vi "Part 1.vi"(11 "Input":string) -> (3 "Output":i64)   [LabVIEW 2021]
uses:
  <userlib>/_OpenG.lib/string/string.llb/Convert EOLs (String)__ogtk.vi
panel:
  out "Array":i64[](array[numeric])
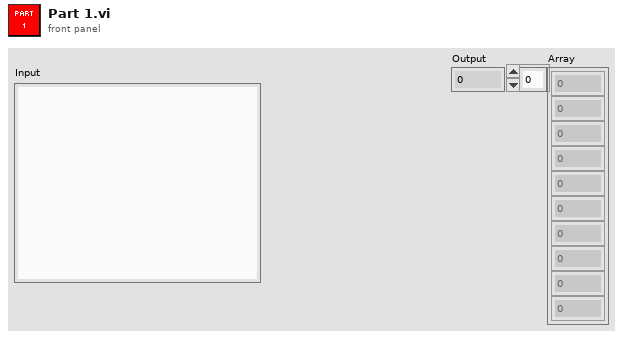
[diagram p1: front panel]
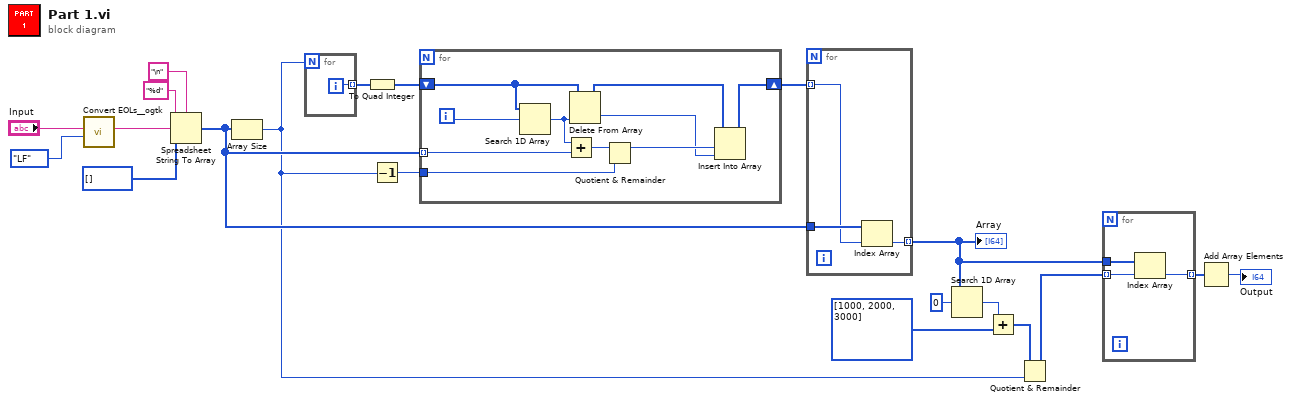
[diagram p0: block diagram]
diagram:
  n1 = call-poly <userlib>:"Convert EOLs__ogtk.vi"("Convert to:"=enum16{"CR", "LF", "CRLF"}."LF", "String in"="Input") -> ("String out"=w16:string)  [unwired: 9 in]
  n2 = Spreadsheet String To Array(delimiter (Tab)="\n", format string="%d", spreadsheet string=w16, array type (2D Dbl)=i64[] []) -> (array=w12:i64[])
  n3 = Array Size(array=w12) -> (size(s)=w8:i32)
  n4 = for {
    N: w8 -> [_]
    tunnel: [w21] -> w7 mode=indexing
    i -> [w21]
  }
  n5 = To Quad Integer(1:w7) -> (0:w6:i64[])
  n6 = Decrement(x=w8) -> (x-1=w14:i32)
  n7 = for {
    tunnel: w12 -> [w31] mode=indexing
    shift-right: [w23] -> w5
    shift-left: w6 -> [w25]
    tunnel: w14 -> [w22]
    i -> [w27]
    n8 = Search 1D Array(1D array=w25, element=w27) -> (index of element=w30:i32)  [unwired: 1 in]
    n9 = Add(x=w30, y=w31) -> (x+y=w29:i64)
    n10 = Delete From Array(array=w25, index=w30) -> (deleted portion=w26:i64, array with subset deleted=w24:i64[])  [unwired: 1 in]
    n11 = Quotient & Remainder(x=w29, y=w22) -> (x-y*floor(x/y)=w28:i64)  [unwired: 1 out]
    n12 = Insert Into Array(array=w24, index=w28, new element=w26) -> (w23:i64[])
  }
  n13 = for {
    tunnel: w5 -> [w33] mode=indexing
    tunnel: w12 -> [w34]
    tunnel: [w32] -> w1 mode=indexing
    n14 = Index Array(array=w34, index=w33) -> (element=w32:i64)
  }
  "Array" <- w1
  n15 = Search 1D Array(1D array=w1, element=i64 0) -> (index of element=w4:i32)  [unwired: 1 in]
  n16 = Add(x=w4, y=i64[] [1000, 2000, 3000]) -> (x+y=w3:i64[])
  n17 = Quotient & Remainder(x=w3, y=w8) -> (x-y*floor(x/y)=w2:i64[])  [unwired: 1 out]
  n18 = for {
    tunnel: w1 -> [w37]
    tunnel: w2 -> [w36] mode=indexing
    tunnel: [w35] -> w10 mode=indexing
    n19 = Index Array(array=w37, index=w36) -> (element=w35:i64)
  }
  n20 = Add Array Elements(numeric array=w10) -> (sum=→"Output":i64)
